vi "SR400 SetDiscParams_a.vi"(6 "error in (no error)":errorcluster, 7 "Discriminateur T":T1 {"Incrément (V)" min=-0.02 max=0.02 step=0.0002; "Niveau (V)" min=-0.3 max=0.3 step=0.0002; "Front A" items=["Montant", "Descendant"]; "Mode" items=["Fixe", "Scan"]}, 8 "Discriminateur A":T1 {"Incrément (V)" min=-0.02 max=0.02 step=0.0002; "Niveau (V)" min=-0.3 max=0.3 step=0.0002; "Front A" items=["Montant", "Descendant"]; "Mode" items=["Fixe", "Scan"]}, 9 "Discriminateur B":T1 {"Incrément (V)" min=-0.02 max=0.02 step=0.0002; "Niveau (V)" min=-0.3 max=0.3 step=0.0002; "Front A" items=["Montant", "Descendant"]; "Mode" items=["Fixe", "Scan"]}, 10 "VISA Port In":refnum<visa-resource-name>="GPIB0::23::INSTR") -> (0 "error out":errorcluster, 3 "VISA Port Out":refnum<visa-resource-name>="GPIB0::23::INSTR")   [LabVIEW 2019]
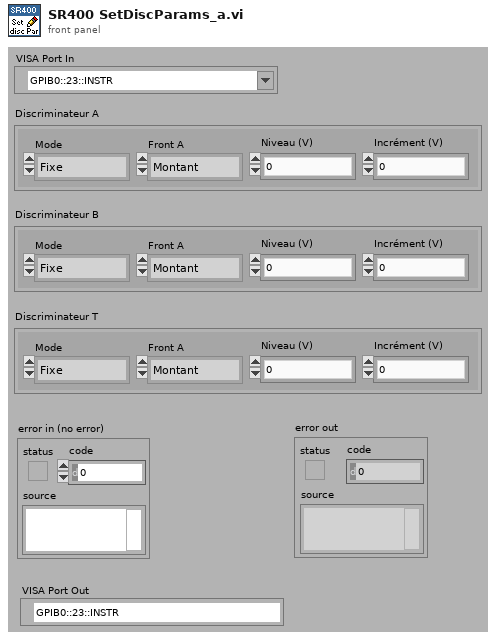
[diagram p1: front panel]
types:
  T1 = cluster{"Mode":u16, "Front A":u16, "Niveau (V)":dbl, "Incrément (V)":dbl}
  T2 = enum16{"Lit le Statut", "Configure", "Oper. incomp."}
  T3 = cluster{"Mode":u16, "Front A":u16, "Niveau (V)":dbl, "Incrément (V)":dbl}[]
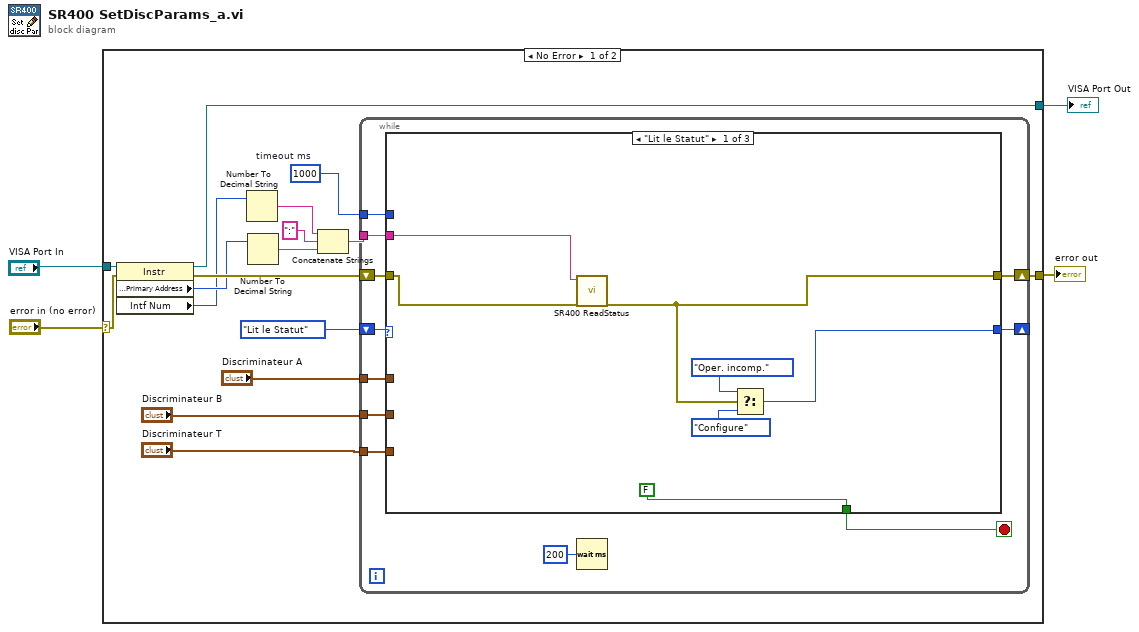
[diagram p0: block diagram]
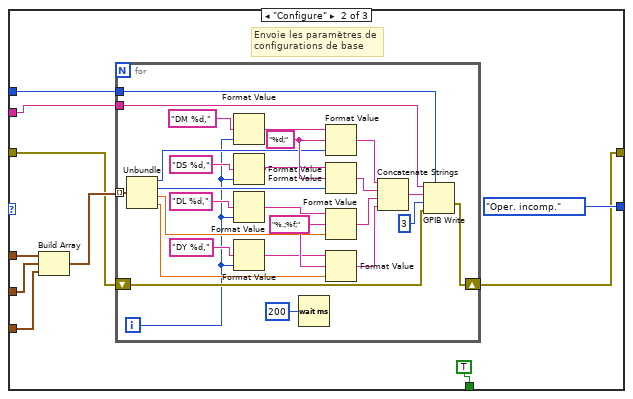
[diagram p2: hidden frame]
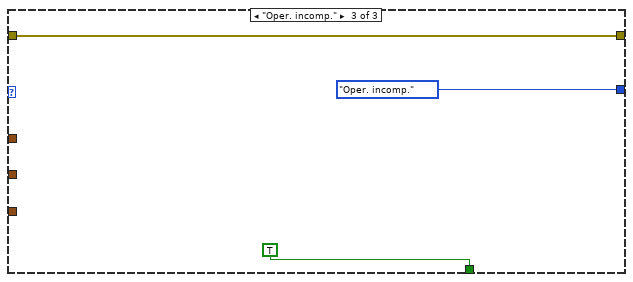
[diagram p3: hidden frame]
diagram:
  n1 = case shown="No Error" "error in (no error)" {
    selector: "error in (no error)" -> [w20 w80]
    tunnel: [w14 w80] -> w3
    tunnel: "VISA Port In" -> [w19 w79]
    tunnel: [w5 w79] -> w1
    frame No Error {
      w15 = 1000  # timeout ms
      n2 = property class="Instr"(reference=w19, error in=w20) -> (reference out=w5:refnum<visa-resource-name>, error out=w18:errorcluster, "GPIB Settings:Primary Address"=w16:u16, "Intf Num"=w10:u16)
      n3 = Number To Decimal String(number=w10) -> (decimal integer string=w7:string)  [unwired: 1 in]
      n4 = Number To Decimal String(number=w16) -> (decimal integer string=w8:string)  [unwired: 1 in]
      n5 = Concatenate Strings(w7, ":" ("string"), w8) -> (w9:string)
      n6 = while {
        shift-right: [w25] -> _
        shift-left: T2."Lit le Statut" -> [w31]
        tunnel: w9 -> [w29]
        shift-right: [w28] -> w14
        shift-left: w18 -> [w30]
        tunnel: w15 -> [w27]
        tunnel: "Discriminateur A" -> [w23]
        tunnel: "Discriminateur B" -> [w22]
        tunnel: "Discriminateur T" -> [w21]
        stop <- w26 stop-if-true
        n7 = case shown="\"Lit le Statut\"" w31 {
          tunnel: w30 -> [w37 w43 w78]
          tunnel: w29 -> [w36 w41 _]
          tunnel: [w32 w39 w78] -> w28
          tunnel: w27 -> [_ w40 _]
          tunnel: [FALSE ("Configuration\neffectuée") TRUE ("Configuration\neffectuée") TRUE ("Configuration\neffectuée")] -> w26
          tunnel: [w33 T2."Oper. incomp." T2."Oper. incomp."] -> w25
          tunnel: w23 -> [_ w47 _]
          tunnel: w22 -> [_ w46 _]
          tunnel: w21 -> [_ w45 _]
          frame "Lit le Statut" {
            n8 = call <userlib>:"SR400 ReadStatus.vi"("error in"=w37, "Address string"=w36) -> ("Error Out"=w32:errorcluster)  [unwired: 6 in, 1 out]
            n9 = Select(t=T2."Oper. incomp.", s=w32, f=T2."Configure") -> (s? t:f=w33:T2)
          }
          frame "Configure" {
            # "Envoie les paramètres de configurations de base"
            n10 = Build Array(w47, w46, w45) -> (w44:T3)
            n11 = for {
              tunnel: w44 -> [w70] mode=indexing
              shift-right: [w54] -> w39
              shift-left: w43 -> [w55]
              tunnel: w41 -> [w53]
              tunnel: w40 -> [w52]
              i -> [w51]
              w68 = "%.;%f;"
              w69 = "%d;"
              n12 = Unbundle(w70) -> ("Mode"=w65:u16, "Front A"=w64:u16, "Niveau (V)"=w63:dbl, "Incrément (V)"=w61:dbl)
              n13 = Format Value(format string="DM %d,", value (0)=w51) -> (output string=w67:string)  [unwired: 1 in]
              n14 = Format Value(format string="DS %d,", value (0)=w51) -> (output string=w66:string)  [unwired: 1 in]
              n15 = Format Value(format string="DL %d,", value (0)=w51) -> (output string=w62:string)  [unwired: 1 in]
              n16 = Format Value(format string="DY %d,", value (0)=w51) -> (output string=w49:string)  [unwired: 1 in]
              n17 = Wait (ms)(milliseconds to wait=u32 200) -> ()  [unwired: 1 out]
              n18 = Format Value(string ("")=w67, format string=w69, value (0)=w65) -> (output string=w60:string)
              n19 = Format Value(string ("")=w66, format string=w69, value (0)=w64) -> (output string=w59:string)
              n20 = Format Value(string ("")=w62, format string=w68, value (0)=w63) -> (output string=w57:string)
              n21 = Format Value(string ("")=w49, format string=w68, value (0)=w61) -> (output string=w58:string)
              n22 = Concatenate Strings(w60, w59, w57, w58) -> (w56:string)
              n23 = GPIB Write(0:w53, 1:w56, 2:i16 3 ("mode (0)"), 3:w55, 4:w52) -> (6:w54:errorcluster)  [unwired: 1 out]
            }
          }
          frame "Oper. incomp." {
          }
        }
        n24 = Wait (ms)(milliseconds to wait=u32 200) -> ()  [unwired: 1 out]
      }
    }
    frame Error {
    }
  }
  "error out" <- w3
  "VISA Port Out" <- w1
